vi "Main.vi"() -> ()   [LabVIEW 2013]
uses:
  source_vi/gui/type_def/device_array.ctl
  source_vi/gui/type_def/device.ctl
  source_vi/gui/type_def/general.ctl
  source_vi/gui/type_def/general_and_device.ctl
  source_vi/queues/que_enqueue_message_single.vi
  source_vi/gui/global_var.vi
panel:
  in  "config_files":string(combo) caption="Configuration file"
  out "log_bar":cluster{u8, u8}(slide) caption="Logging" scale=10.0..100.0
  out "srv_bar":cluster{u8, u8}(slide) caption="Server" scale=10.0..100.0
  in  "logging?":bool
  in  "gral_&-device":T1={"general"={"file_ext"="0.0.0.0", "TCP port"=0, "#devices"=0, "log?"=FALSE, "tcp?"=FALSE, "language"="ENG"}, "eeg_device"={"name"="", "hardware"="", "image"="", "path"=path "", "extra"="", "channels"=""}}
  out "eeg_device":T3
  in  "serving?":bool
  in  "acquiring?":bool
  in  "stopBars":bool
  out "acq_bar":cluster{u8, u8}(slide) caption="Acquistion" scale=10.0..100.0
  in  "log?":bool caption="Save Log"
  in  "tcp?":bool caption="Save Log"
  in  "refuse mrk?":bool
  out "images":picture[](array[picture])
  out "general":T2={"file_ext"="CSV", "TCP port"=0, "#devices"=0, "log?"=FALSE, "tcp?"=FALSE, "language"="ENG"}
  out "devices":T4
  in  "play?":bool
  out "log_box":string
  in  "stop?":bool
  in  "eeg_txtbox":string(combo) caption="Device"
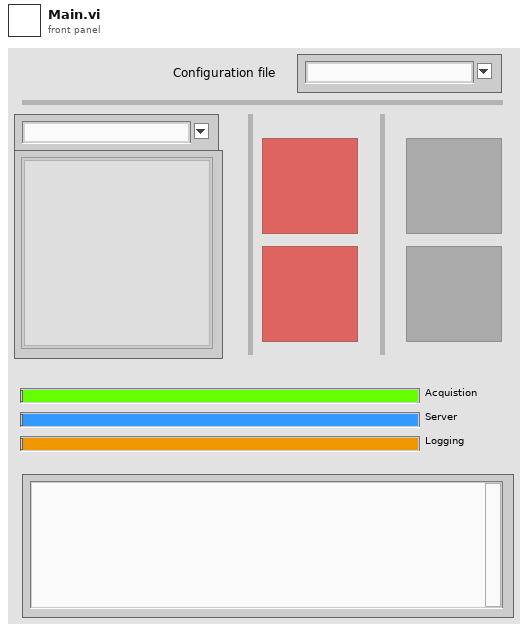
[diagram p1: front panel]
types:
  T1 = typedef "general_and_device.ctl" = cluster{"general":T2, "eeg_device":T3}
  T2 = typedef "general.ctl" = cluster{"file_ext":string, "TCP port":i32, "#devices":i32, "log?":bool, "tcp?":bool, "language":string}
  T3 = typedef "device.ctl" = cluster{"name":string, "hardware":string, "image":string, "path":path, "extra":string, "channels":string}
  T4 = typedef "device_array.ctl" = T3[]
  T5 = typedef "que_all_message_queues.ctl" = cluster{"UI":refnum<queue>, "Acquisition":refnum<queue>, "Server":refnum<queue>, "Logging":refnum<queue>}
  T6 = typedef "imagedata.ctl" = cluster{"image type":i32, "image depth":i32, "image":u8[], "mask":u8[], "colors":u32[], "Rectangle":cluster{"left":i16, "top":i16, "right":i16, "bottom":i16}}
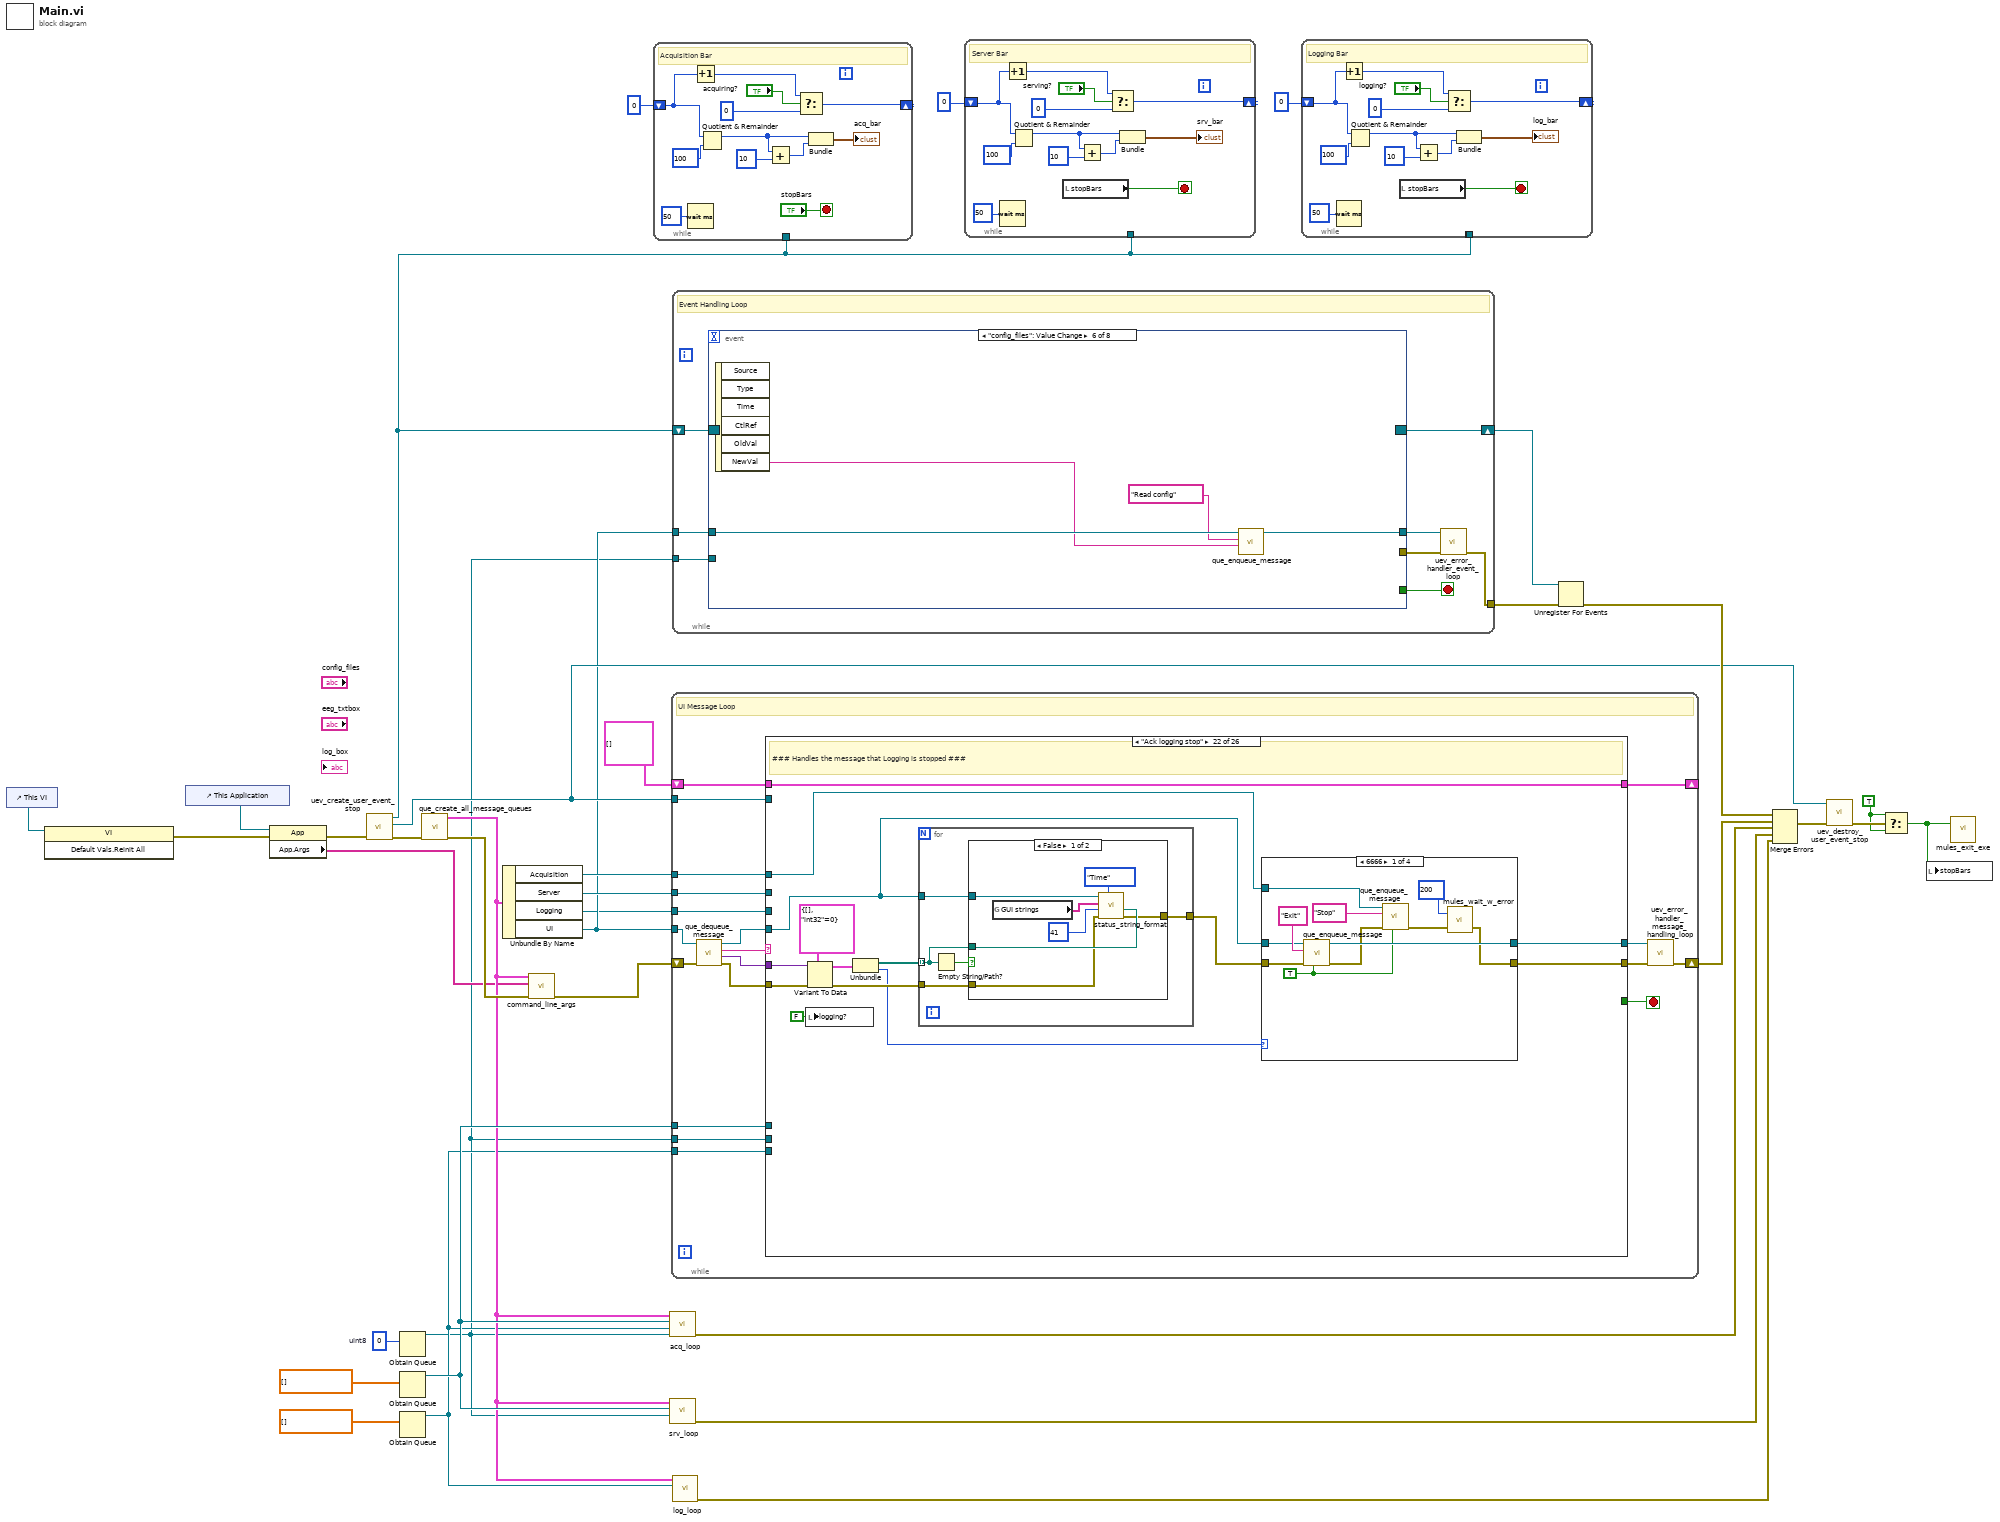
[diagram p0: block diagram]
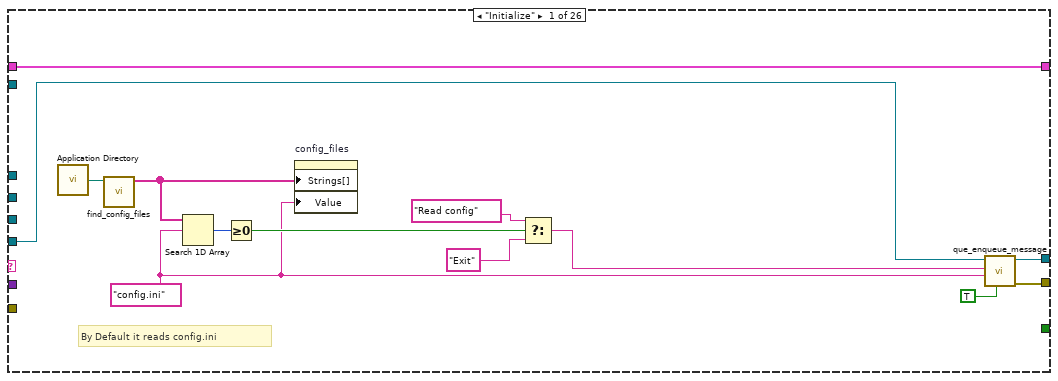
[diagram p2: hidden frame]
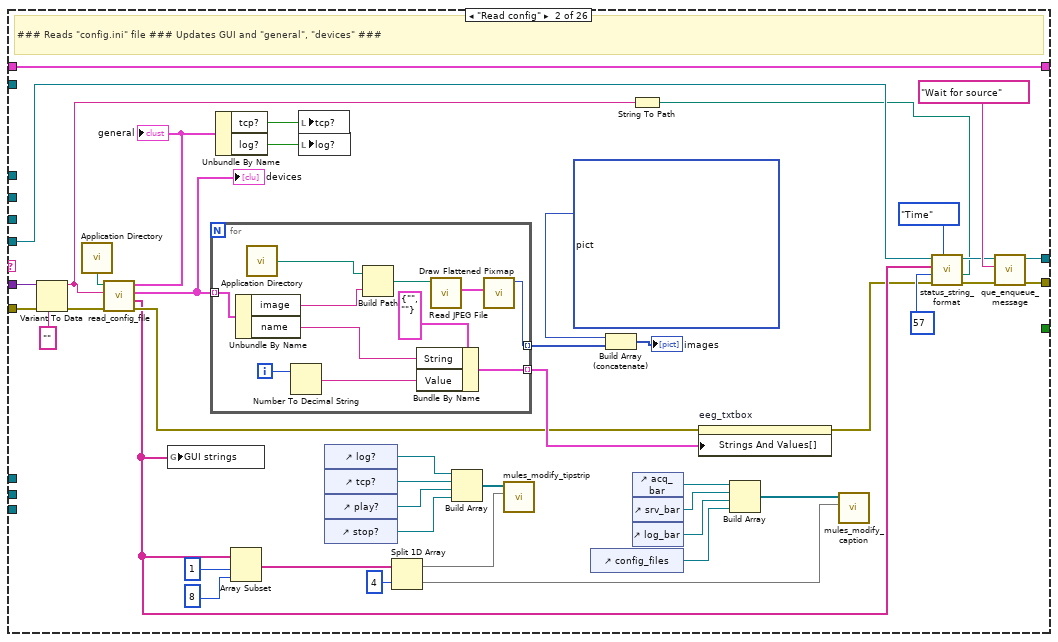
[diagram p3: hidden frame]
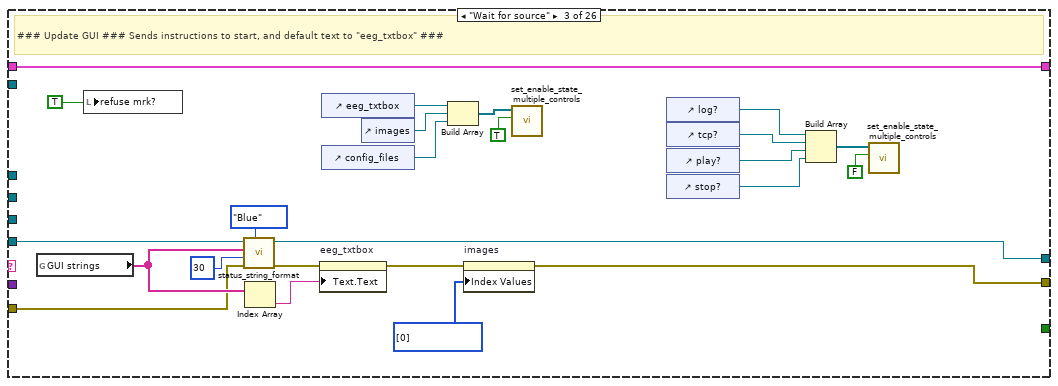
[diagram p4: hidden frame]
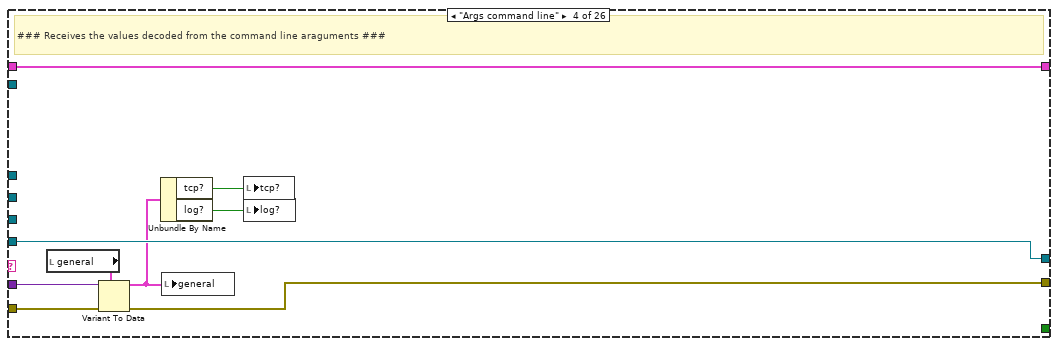
[diagram p5: hidden frame]
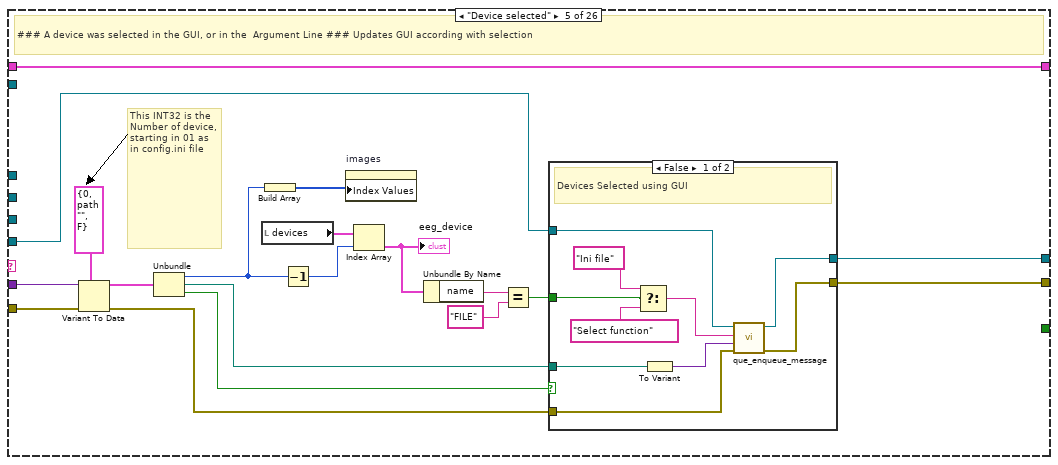
[diagram p6: hidden frame]
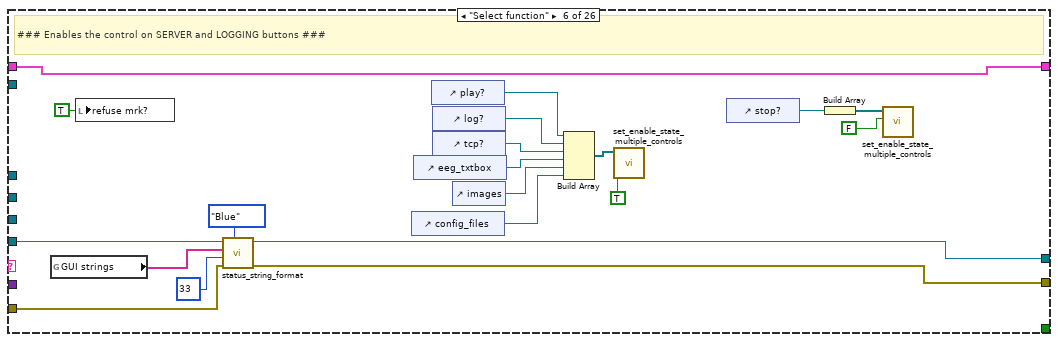
[diagram p8: hidden frame]
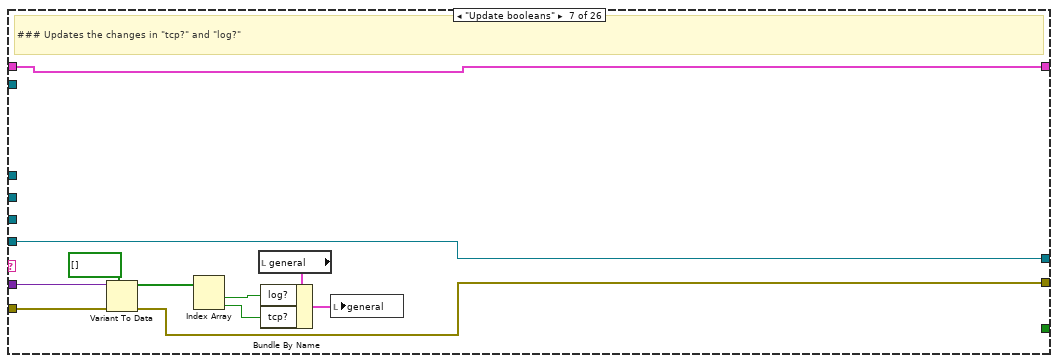
[diagram p9: hidden frame]
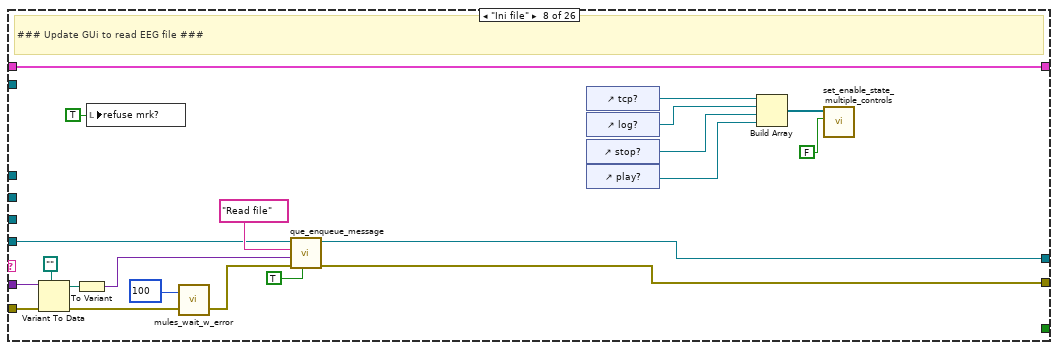
[diagram p10: hidden frame]
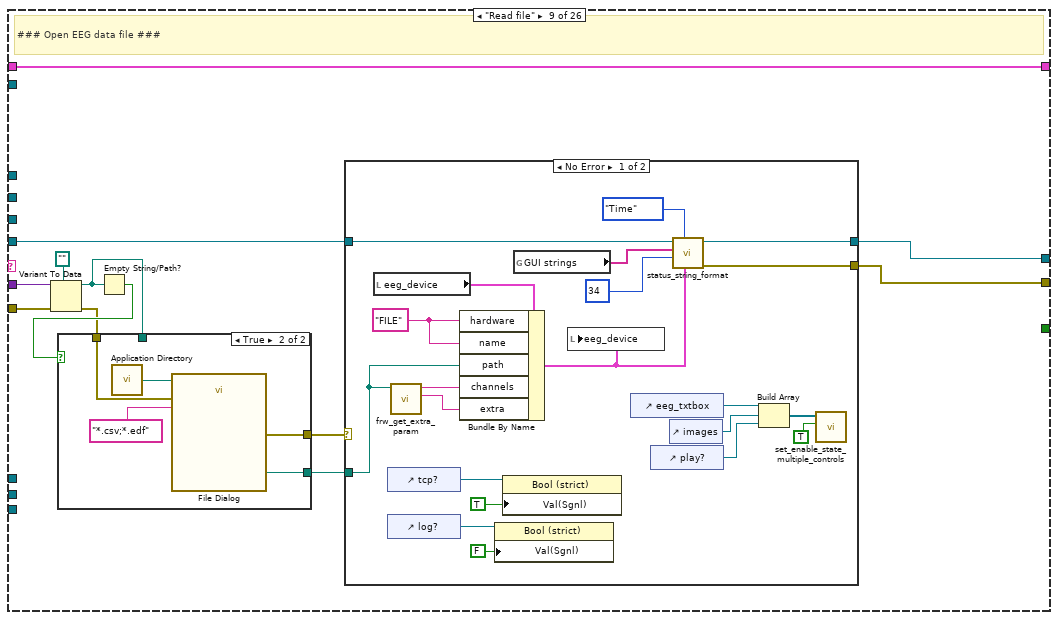
[diagram p11: hidden frame]
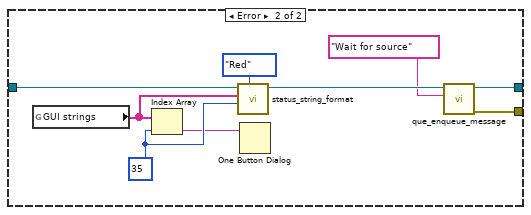
[diagram p13: hidden frame]
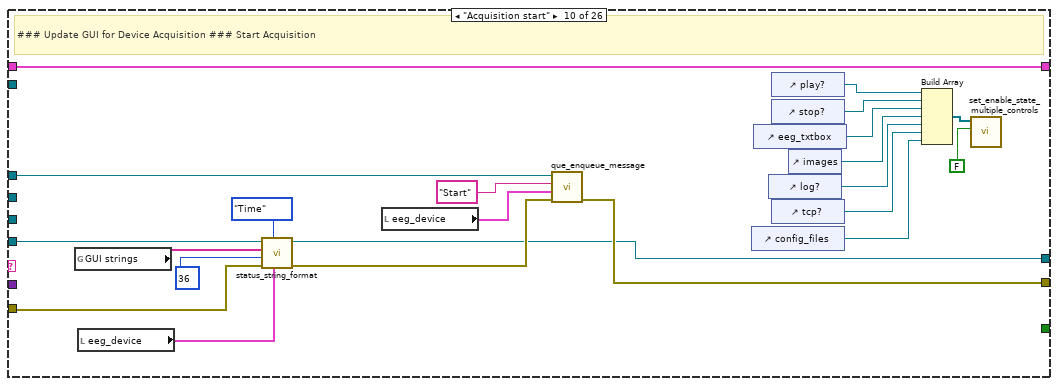
[diagram p14: hidden frame]
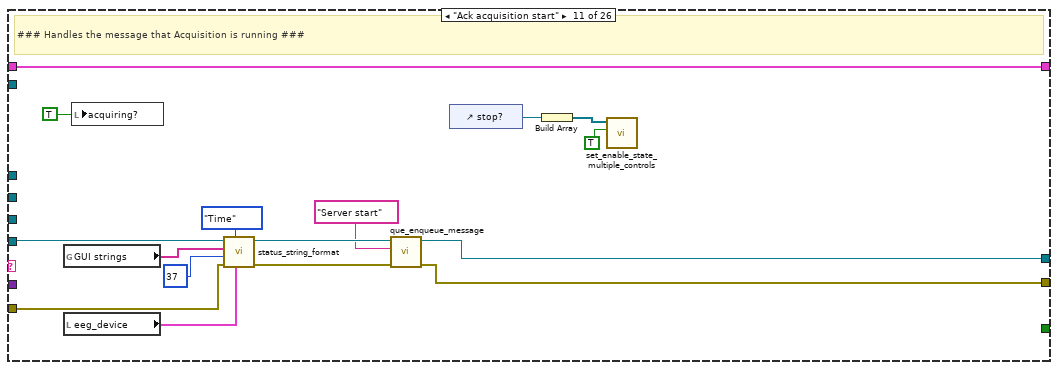
[diagram p15: hidden frame]
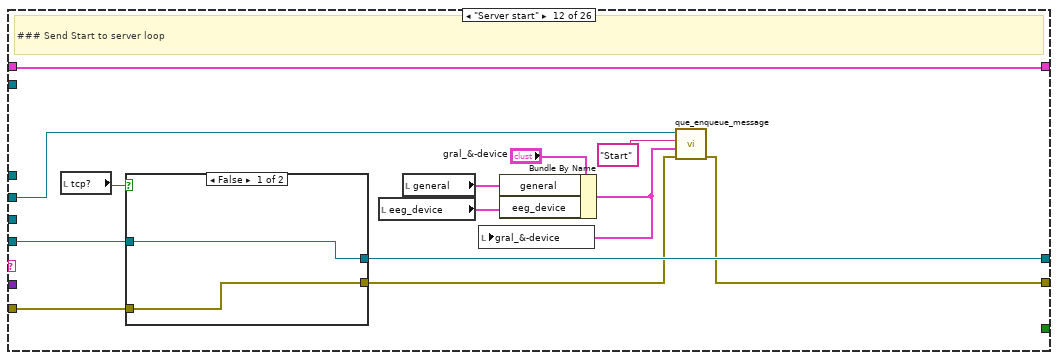
[diagram p16: hidden frame]
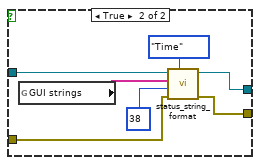
[diagram p17: hidden frame]
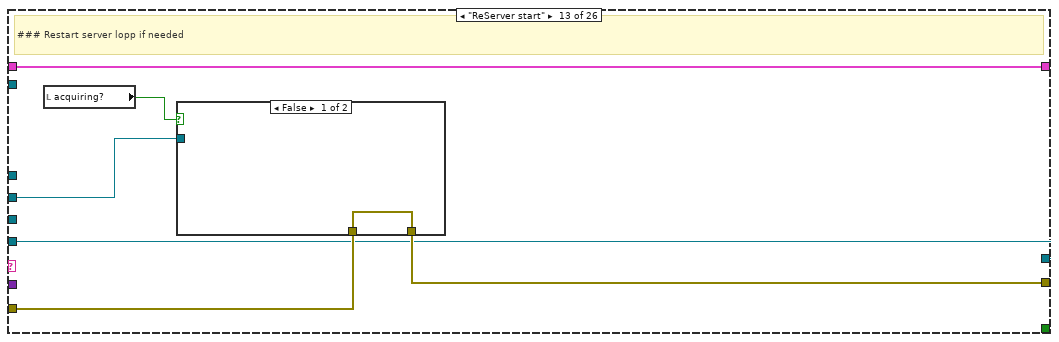
[diagram p18: hidden frame]
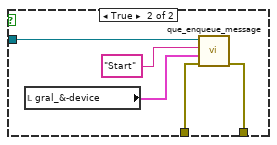
[diagram p19: hidden frame]
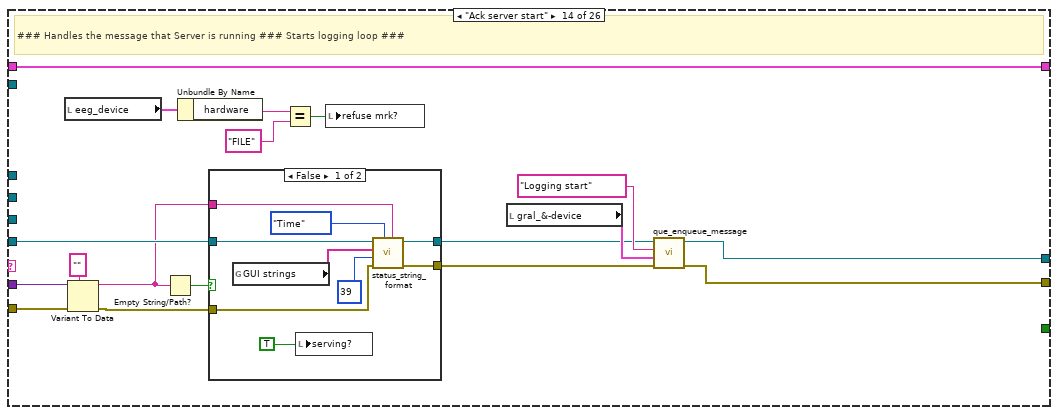
[diagram p20: hidden frame]
diagram:
  w20 = TRUE
  w27 = u8 0  # uint8
  n1 = control-ref of="This VI"() -> (w28:refnum<vi>)
  n2 = invoke class="VI" method="Default Vals.Reinit All"(reference=w28) -> (error out=w10:errorcluster)  [unwired: 2 in, 2 out]
  n3 = control-ref of="This Application"() -> (w12:refnum<vi>)
  n4 = property class="App"(reference=w12, error in=w10) -> (error out=w11:errorcluster, "App.Args"=w6:string[])  [unwired: 1 out]
  n5 = call "uev_create_user_event_stop.vi"("error in (no error)"=w11) -> ("error out"=w23:errorcluster, "User Event - Stop"=w31:refnum<user-event>, "Stop Event Registration Refnum"=w4:refnum<event-registration>)  [unwired: 8 in]
  n6 = Obtain Queue(element data type=w27) -> (queue out=w1:refnum<queue>)  [unwired: 4 in, 2 out]
  n7 = Obtain Queue(element data type=dbl[] []) -> (queue out=w16:refnum<queue>)  [unwired: 4 in, 2 out]
  n8 = Obtain Queue(element data type=dbl[] []) -> (queue out=w2:refnum<queue>)  [unwired: 4 in, 2 out]
  n9 = call "que_create_all_message_queues.vi"("error in (no error)"=w23) -> ("error out"=w8:errorcluster, "Message Queues out"=w7:T5)  [unwired: 9 in]
  n10 = Unbundle By Name(w7) -> ("Acquisition"=w30:refnum<queue>, "Server"=w29:refnum<queue>, "Logging"=w18:refnum<queue>, "UI"=w19:refnum<queue>)
  n11 = call "command_line_args.vi"("error in (no error)"=w8, "App.Args"=w6, "Message Queues"=w7) -> ("error out"=w9:errorcluster)  [unwired: 7 in, 1 out]
  n12 = while {
    shift-right: [w40] -> _
    shift-left: 0 ("y") -> [w42]
    tunnel: w4 -> [_]
    stop <- "stopBars" stop-if-true
    # "Acquisition Bar"
    n13 = Wait (ms)(milliseconds to wait=u32 50 ("millisecond multiple")) -> ()  [unwired: 1 out]
    n14 = Increment(x=w42) -> (x+1=w41:i32)
    n15 = Quotient & Remainder(x=w42, y=100) -> (x-y*floor(x/y)=w45:i32)  [unwired: 1 out]
    n16 = Add(x=w45, y=u32 10 ("millisecond multiple")) -> (x+y=w48:u32)
    n17 = Select(t=w41, s="acquiring?", f=0 ("y")) -> (s? t:f=w40:i32)
    n18 = Bundle(w45, w48) -> (→"acq_bar":cluster{i32, u32})  [unwired: 1 in]
  }
  n19 = call "acq_loop.vi"("Marker Queue"=w1, "Log queue"=w2, "Server queue"=w16, "Message Queues"=w7) -> ("error out"=w22:errorcluster)  [unwired: 7 in]
  n20 = call "srv_loop.vi"("Marker Queue"=w1, "Server queue"=w16, "Message Queues"=w7) -> ("error out"=w17:errorcluster)  [unwired: 8 in]
  n21 = while {
    tunnel: w19 -> [w66]
    shift-right: [w54] -> w32
    shift-left: w9 -> [w67]
    tunnel: w29 -> [w61]
    tunnel: w31 -> [w60]
    tunnel: w30 -> [w59]
    tunnel: w16 -> [w52]
    tunnel: w1 -> [w57]
    shift-right: [w55] -> _
    shift-left: cluster{"String":string, "Color Box":u32}[] [] -> [w56]
    tunnel: w18 -> [w53]
    tunnel: w2 -> [w50]
    stop <- w58 stop-if-true
    # "UI Message Loop"
    n22 = call "que_dequeue_message.vi"("error in (no error)"=w67, "Message Queue"=w66) -> ("error out"=w65:errorcluster, "Message Data"=w64:variant, "Message"=w49:string, "dup Message Queue"=w63:refnum<queue>)  [unwired: 6 in]
    n23 = case shown="\"Ack logging stop\"" w49 {
      selector: w49 -> [_ _ _ _ _ _ _ _ _ _ _ _ _ _ _ _ _ _ _ _ _ _ _ _ _ w701]
      tunnel: w65 -> [_ w95 w137 w164 w168 w202 w221 w235 w252 w315 w327 w342 w363 w386 w404 w415 w438 w456 w485 w508 w532 w558 w607 w666 w693 w714]
      tunnel: w64 -> [_ w96 _ w167 w181 _ w227 w236 w255 _ _ _ _ w388 _ w416 w436 w459 w484 w512 w531 w560 w622 _ w692 _]
      tunnel: w63 -> [w75 w88 w156 w162 w178 w209 w219 w238 w262 w320 w333 w345 w361 w385 w402 w412 w444 w453 w477 w509 w528 w550 _ w663 w691 w715]
      tunnel: [w80 w91 w140 w163 w177 w201 w220 w240 w257 w310 w329 w338 w362 w379 w403 w411 w440 w461 w487 w506 w530 w548 w608 w665 w690 w703] -> w62
      tunnel: w61 -> [_ _ _ _ _ _ _ _ _ _ _ w341 w364 _ _ _ _ _ w488 _ _ _ _ _ _ w712]
      tunnel: w60 -> [_ _ _ _ _ _ _ _ _ _ _ _ _ _ _ _ _ _ _ _ _ _ _ _ _ w713]
      tunnel: w59 -> [_ _ _ _ _ _ _ _ _ w312 _ _ _ _ _ _ w442 _ _ _ _ w547 _ _ _ w711]
      tunnel: [_ _ _ _ _ _ _ _ _ _ _ _ _ _ _ _ _ _ _ _ _ _ _ _ _ TRUE ("Discard?")] -> w58
      tunnel: w52 -> [_ _ _ _ _ _ _ _ _ _ _ _ _ _ _ _ _ _ _ _ _ _ _ _ _ w708]
      tunnel: w57 -> [_ _ _ _ _ _ _ _ _ _ _ _ _ _ _ _ _ _ _ _ _ _ _ _ _ w707]
      tunnel: w56 -> [w78 w116 w139 w165 w172 w214 w222 w245 w261 w321 w323 w350 w365 w389 w401 w409 w449 w475 w490 w513 w537 w559 w620 w669 w689 w699]
      tunnel: [w78 w116 w139 w165 w172 w214 w222 w245 w261 w321 w323 w350 w365 w389 w401 w409 w449 w475 w490 w513 w537 w559 w613 w669 w689 w699] -> w55
      tunnel: w53 -> [_ _ _ _ _ _ _ _ _ _ _ _ _ _ w405 _ _ _ _ _ w524 _ _ _ _ w700]
      tunnel: [w79 w90 w136 w162 w176 w200 w219 w239 w258 w309 w328 w343 w361 w372 w402 w410 w443 w457 w478 w505 w525 w549 _ w664 w686 _] -> w51
      tunnel: w50 -> [_ _ _ _ _ _ _ _ _ _ _ _ _ _ _ _ _ _ _ _ _ _ _ _ _ w704]
      frame "Initialize" {
        w70 = "config.ini" ("Message")
        # "By Default it reads config.ini"
        n24 = call <vilib>:"Application Directory.vi"() -> ("Application Directory"=w76:path)
        n25 = call "find_config_files.vi"("path"=w76) -> ("config files_names"=w73:string[])  [unwired: 10 in]
        n26 = Search 1D Array(1D array=w73, element=w70) -> (index of element=w74:i32)  [unwired: 1 in]
        n27 = Greater Or Equal To 0?(x=w74) -> (x >= 0?=w71:bool)
        n28 = property on="config_files" class="CmbBox"("Strings[]"=w73, "Value"=w70) -> ()  [unwired: 2 in, 2 out]
        n29 = Select(t="Read config" ("Message"), s=w71, f="Exit" ("Message")) -> (s? t:f=w72:string)
        n30 = call-poly "que_enqueue_message.vi"("Priority Message? (F)"=TRUE, "Message Data"=w70, "Message"=w72, "Message Queue"=w75) -> ("error out"=w80:errorcluster, "dup Message Queue"=w79:refnum<queue>)  [unwired: 6 in]
      }
      frame "Read config" {
        # "### Reads \"config.ini\" file ### Updates GUI and \"general\", \"devices\" ###"
        n31 = Variant To Data(error in=w95, type="", Variant=w96) -> (data=w85:string, error out=w94:errorcluster)
        n32 = call <vilib>:"Application Directory.vi"() -> ("Application Directory"=w98:path)
        n33 = call "read_config_file.vi"("error in (no error)"=w94, "filename"=w85, "Application Directory"=w98) -> ("error out"=w115:errorcluster, "gui_strings"=w86:string[], "devices"=w117:T4, "gral_config"=w123:T2)  [unwired: 5 in]
        "devices" <- w117
        "general" <- w123
        n34 = global write "global_var.vi" "GUI strings"(w86) -> ()
        n35 = for {
          tunnel: w117 -> [w134] mode=indexing
          tunnel: [w132] -> w121 mode=indexing
          tunnel: [w128] -> w122 mode=indexing
          i -> [w131]
          n36 = Unbundle By Name(w134) -> ("image"=w124:string, "name"=w127:string)
          n37 = call <vilib>:"Application Directory.vi"() -> ("Application Directory"=w125:path)
          n38 = Number To Decimal String(number=w131) -> (decimal integer string=w129:string)  [unwired: 1 in]
          n39 = Build Path(base path=w125, name or relative path=w124) -> (appended path=w126:path)
          n40 = Bundle By Name(cluster=cluster{"String":string, "Value":string} {"String"="", "Value"=""} ("element"), "String"=w127, "Value"=w129) -> (w128:cluster{"String":string, "Value":string})
          n41 = call <vilib>:"Read JPEG File.vi"("path to JPEG file"=w126) -> ("image data"=w133:T6)  [unwired: 8 in, 2 out]
          n42 = call <vilib>:"Draw Flattened Pixmap.vi"("image data"=w133) -> ("new picture"=w132:picture)  [unwired: 8 in]
        }
        n43 = Unbundle By Name(w123) -> ("tcp?"=w119:bool, "log?"=w118:bool)
        n44 = Array Subset(array=w86, index=1, length=8) -> (w103:string[])
        n45 = local write "tcp?"(w119) -> ()
        n46 = local write "log?"(w118) -> ()
        n47 = control-ref of="log?"() -> (w112:refnum<vi>)
        n48 = control-ref of="tcp?"() -> (w111:refnum<vi>)
        n49 = control-ref of="play?"() -> (w110:refnum<vi>)
        n50 = control-ref of="stop?"() -> (w109:refnum<vi>)
        n51 = Split 1D Array(array=w103, index=4) -> (first subarray=w101:string[], second subarray=w100:string[])
        n52 = Build Array(w112, w111, w110, w109) -> (w108:refnum<vi>[])
        n53 = call "mules_modify_tipstrip.vi"("Tip Strip Array"=w101, "Controls"=w108) -> ()  [unwired: 10 in]
        n54 = control-ref of="config_files"() -> (w93:refnum<vi>)
        n55 = Build Array (concatenate)(picture bytes[110622] ("2D Picture"), w121) -> (→"images":picture[])
        n56 = String To Path(string=w85) -> (path=w84:path)
        n57 = control-ref of="acq_bar"() -> (w107:refnum<vi>)
        n58 = control-ref of="srv_bar"() -> (w106:refnum<vi>)
        n59 = control-ref of="log_bar"() -> (w105:refnum<vi>)
        n60 = property on="eeg_txtbox" class="CmbBox"(error in=w115, "Strings And Values[]"=w122) -> (error out=w81:errorcluster)  [unwired: 1 in, 1 out]
        n61 = Build Array(w107, w106, w105, w93) -> (w104:refnum<vi>[])
        n62 = call "mules_modify_caption.vi"("Tip Strip Array"=w100, "Controls"=w104) -> ()  [unwired: 10 in]
        n63 = call "status_string_format.vi"("log_file"=w84, "color"=enum16{"Black", "Blue", "Red", "Time"}."Time", "error in (no error)"=w81, "index"=57, "gui_strings"=w86, "Message Queue"=w88) -> ("error out"=w87:errorcluster, "dup Message Queue"=w89:refnum<queue>)  [unwired: 4 in]
        n64 = call-poly "que_enqueue_message.vi"("error in (no error)"=w87, "Message"="Wait for source", "Message Queue"=w89) -> ("error out"=w91:errorcluster, "dup Message Queue"=w90:refnum<queue>)  [unwired: 7 in]
      }
      frame "Wait for source" {
        # "### Update GUI ### Sends instructions to start, and default text to \"eeg_txtbox\" ###"
        n65 = global read "global_var.vi" "GUI strings"() -> (w138:string[])
        n66 = local write "refuse mrk?"(TRUE) -> ()
        n67 = call "status_string_format.vi"("color"=enum16{"Black", "Blue", "Red", "Time"}."Blue", "error in (no error)"=w137, "index"=30, "gui_strings"=w138, "Message Queue"=w156) -> ("error out"=w152:errorcluster, "dup Message Queue"=w136:refnum<queue>)  [unwired: 5 in]
        n68 = Index Array(array=w138) -> (element=w153:string)  [unwired: 1 in]
        n69 = property on="eeg_txtbox" class="CmbBox"(error in=w152, "Text.Text"=w153) -> (error out=w155:errorcluster)  [unwired: 1 in, 1 out]
        n70 = control-ref of="eeg_txtbox"() -> (w144:refnum<vi>)
        n71 = control-ref of="config_files"() -> (w135:refnum<vi>)
        n72 = control-ref of="images"() -> (w143:refnum<vi>)
        n73 = Build Array(w144, w143, w135) -> (w141:refnum<vi>[])
        n74 = property on="images" class="Arr (strict)"(error in=w155, "Index Values"=u32[] [0]) -> (error out=w140:errorcluster)  [unwired: 1 in, 1 out]
        n75 = call "set_enable_state_multiple_controls.vi"("Enable?"=TRUE, "Controls"=w141) -> ()  [unwired: 10 in]
        n76 = control-ref of="log?"() -> (w145:refnum<vi>)
        n77 = control-ref of="tcp?"() -> (w146:refnum<vi>)
        n78 = control-ref of="play?"() -> (w147:refnum<vi>)
        n79 = control-ref of="stop?"() -> (w148:refnum<vi>)
        n80 = Build Array(w145, w146, w147, w148) -> (w151:refnum<vi>[])
        n81 = call "set_enable_state_multiple_controls.vi"("Enable?"=FALSE, "Controls"=w151) -> ()  [unwired: 10 in]
      }
      frame "Args command line" {
        # "### Receives the values decoded from the command line araguments ###"
        n82 = local read "general"() -> (w166:T2)
        n83 = Variant To Data(error in=w164, type=w166, Variant=w167) -> (data=w159:T2, error out=w163:errorcluster)
        n84 = Unbundle By Name(w159) -> ("tcp?"=w161:bool, "log?"=w160:bool)
        n85 = local write "general"(w159) -> ()
        n86 = local write "tcp?"(w161) -> ()
        n87 = local write "log?"(w160) -> ()
      }
      frame "Device selected" {
        # "This INT32 is the Number of device, starting in 01 as in config.ini file"
        # "### A device was selected in the GUI, or in the  Argument Line ### Updates GUI according with selection"
        n88 = Variant To Data(error in=w168, type=cluster{i32, path, bool} {0, path "", FALSE} ("output cluster"), Variant=w181) -> (data=w175:cluster{i32, path, bool}, error out=w169:errorcluster)
        n89 = Unbundle(w175) -> (w174:i32, w173:path, w170:bool)
        n90 = local read "devices"() -> (w182:T4)
        n91 = Build Array(w174) -> (w180:i32[])
        n92 = Decrement(x=w174) -> (x-1=w179:i32)
        n93 = property on="images" class="Arr (strict)"("Index Values"=w180) -> ()  [unwired: 2 in, 2 out]
        n94 = Index Array(array=w182, index=w179) -> (element=w183:T3)
        "eeg_device" <- w183
        n95 = Unbundle By Name(w183) -> ("name"=w184:string)
        n96 = Equal?(x=w184, y="FILE" ("Message")) -> (x = y?=w186:bool)
        n97 = case shown="False" w170 {
          tunnel: w186 -> [w193 _]
          tunnel: w178 -> [w192 w198]
          tunnel: [w191 w197] -> w177
          tunnel: [w190 w198] -> w176
          tunnel: w173 -> [w189 _]
          tunnel: w169 -> [w187 w197]
          frame False {
            # "Devices Selected using GUI"
            n98 = Select(t="Ini file" ("Message"), s=w193, f="Select function" ("Message")) -> (s? t:f=w196:string)
            n99 = To Variant(anything=w189) -> (Variant=w188:variant)
            n100 = call-poly "que_enqueue_message.vi"("error in (no error)"=w187, "Message Data"=w188, "Message"=w196, "Message Queue"=w192) -> ("error out"=w191:errorcluster, "dup Message Queue"=w190:refnum<queue>)  [unwired: 6 in]
          }
          frame True {
            # "Device Selected in Argument Line"
          }
        }
      }
      frame "Select function" {
        # "### Enables the control on SERVER and LOGGING buttons ###"
        n101 = global read "global_var.vi" "GUI strings"() -> (w208:string[])
        n102 = local write "refuse mrk?"(TRUE) -> ()
        n103 = call "status_string_format.vi"("color"=enum16{"Black", "Blue", "Red", "Time"}."Blue", "error in (no error)"=w202, "index"=33, "gui_strings"=w208, "Message Queue"=w209) -> ("error out"=w201:errorcluster, "dup Message Queue"=w200:refnum<queue>)  [unwired: 5 in]
        n104 = control-ref of="config_files"() -> (w199:refnum<vi>)
        n105 = control-ref of="eeg_txtbox"() -> (w211:refnum<vi>)
        n106 = control-ref of="play?"() -> (w203:refnum<vi>)
        n107 = control-ref of="log?"() -> (w204:refnum<vi>)
        n108 = control-ref of="tcp?"() -> (w205:refnum<vi>)
        n109 = control-ref of="images"() -> (w210:refnum<vi>)
        n110 = Build Array(w203, w204, w205, w211, w210, w199) -> (w213:refnum<vi>[])
        n111 = call "set_enable_state_multiple_controls.vi"("Enable?"=TRUE, "Controls"=w213) -> ()  [unwired: 10 in]
        n112 = control-ref of="stop?"() -> (w218:refnum<vi>)
        n113 = Build Array(w218) -> (w217:refnum<vi>[])
        n114 = call "set_enable_state_multiple_controls.vi"("Enable?"=FALSE, "Controls"=w217) -> ()  [unwired: 10 in]
      }
      frame "Update booleans" {
        # "### Updates the changes in \"tcp?\" and \"log?\""
        n115 = Variant To Data(error in=w221, type=bool[] [], Variant=w227) -> (data=w225:bool[], error out=w220:errorcluster)
        n116 = Index Array(array=w225) -> (element #1=w224:bool, element #2=w223:bool)  [unwired: 2 in]
        n117 = local read "general"() -> (w228:T2)
        n118 = Bundle By Name(cluster=w228, "log?"=w224, "tcp?"=w223) -> (w229:T2)
        n119 = local write "general"(w229) -> ()
      }
      frame "Ini file" {
        # "### Update GUi to read EEG file ###"
        n120 = Variant To Data(error in=w235, type=path "", Variant=w236) -> (data=w232:path, error out=w234:errorcluster)
        n121 = To Variant(anything=w232) -> (Variant=w231:variant)
        n122 = local write "refuse mrk?"(TRUE) -> ()
        n123 = call "mules_wait_w_error.vi"("error in (no error)"=w234, "milliseconds to wait"=u32 100) -> ("error out"=w242:errorcluster)  [unwired: 1 in]
        n124 = call-poly "que_enqueue_message.vi"("Priority Message? (F)"=TRUE, "error in (no error)"=w242, "Message Data"=w231, "Message"="Read file", "Message Queue"=w238) -> ("error out"=w240:errorcluster, "dup Message Queue"=w239:refnum<queue>)  [unwired: 5 in]
        n125 = control-ref of="tcp?"() -> (w237:refnum<vi>)
        n126 = control-ref of="log?"() -> (w244:refnum<vi>)
        n127 = control-ref of="stop?"() -> (w250:refnum<vi>)
        n128 = control-ref of="play?"() -> (w249:refnum<vi>)
        n129 = Build Array(w237, w244, w250, w249) -> (w248:refnum<vi>[])
        n130 = call "set_enable_state_multiple_controls.vi"("Enable?"=FALSE, "Controls"=w248) -> ()  [unwired: 10 in]
      }
      frame "Read file" {
        # "### Open EEG data file ###"
        n131 = Variant To Data(error in=w252, type=path "", Variant=w255) -> (data=w253:path, error out=w251:errorcluster)
        n132 = Empty String/Path?(string/path=w253) -> (empty?=w254:bool)
        n133 = case shown="True" w254 {
          tunnel: [w263 w269] -> w260
          tunnel: [w264 w268] -> w259
          tunnel: w253 -> [w264 _]
          tunnel: w251 -> [w263 w267]
          frame False {
          }
          frame True {
            n134 = call <vilib>:"Application Directory.vi"() -> ("Application Directory"=w265:path)
            n135 = call "File Dialog"("start path"=w265, "error in"=w267, "pattern (all files)"="*.csv;*.edf") -> ("selected path"=w268:path, "error out"=w269:errorcluster)  [unwired: 9 in, 2 out]
          }
        }
        n136 = case shown="No Error" w260 {
          tunnel: w262 -> [w286 w299]
          tunnel: w259 -> [w283 _]
          tunnel: [w287 w294] -> w258
          tunnel: [w279 w292] -> w257
          frame No Error {
            w280 = "FILE" ("Message")
            n137 = local read "eeg_device"() -> (w290:T3)
            n138 = control-ref of="tcp?"() -> (w270:refnum<vi>)
            n139 = control-ref of="log?"() -> (w273:refnum<vi>)
            n140 = call "frw_get_extra_param.vi"("Path"=w283) -> ("extra_string"=w281:string, "channels_str"=w282:string)  [unwired: 9 in]
            n141 = Bundle By Name(cluster=w290, "hardware"=w280, "name"=w280, "path"=w283, "channels"=w282, "extra"=w281) -> (w285:T3)
            n142 = property class="Bool (strict)"(reference=w273, "Val(Sgnl)"=FALSE ("Value (Signaling)")) -> ()  [unwired: 1 in, 2 out]
            n143 = property class="Bool (strict)"(reference=w270, "Val(Sgnl)"=TRUE ("Value (Signaling)")) -> ()  [unwired: 1 in, 2 out]
            n144 = global read "global_var.vi" "GUI strings"() -> (w289:string[])
            n145 = local write "eeg_device"(w285) -> ()
            n146 = control-ref of="eeg_txtbox"() -> (w275:refnum<vi>)
            n147 = control-ref of="play?"() -> (w277:refnum<vi>)
            n148 = control-ref of="images"() -> (w274:refnum<vi>)
            n149 = call "status_string_format.vi"("eeg_device"=w285, "color"=enum16{"Black", "Blue", "Red", "Time"}."Time", "index"=34, "gui_strings"=w289, "Message Queue"=w286) -> ("error out"=w279:errorcluster, "dup Message Queue"=w287:refnum<queue>)  [unwired: 5 in]
            n150 = Build Array(w275, w274, w277) -> (w276:refnum<vi>[])
            n151 = call "set_enable_state_multiple_controls.vi"("Enable?"=TRUE, "Controls"=w276) -> ()  [unwired: 10 in]
          }
          frame Error {
            w297 = 35 ("index")
            n152 = global read "global_var.vi" "GUI strings"() -> (w298:string[])
            n153 = Index Array(array=w298, index=w297) -> (element=w291:string)
            n154 = call "status_string_format.vi"("color"=enum16{"Black", "Blue", "Red", "Time"}."Red", "index"=w297, "gui_strings"=w298, "Message Queue"=w299) -> ("dup Message Queue"=w295:refnum<queue>)  [unwired: 6 in, 1 out]
            n155 = One Button Dialog(message=w291) -> ()  [unwired: 1 in, 1 out]
            n156 = call-poly "que_enqueue_message.vi"("Message"="Wait for source", "Message Queue"=w295) -> ("error out"=w292:errorcluster, "dup Message Queue"=w294:refnum<queue>)  [unwired: 8 in]
          }
        }
      }
      frame "Acquisition start" {
        # "### Update GUI for Device Acquisition ### Start Acquisition"
        n157 = global read "global_var.vi" "GUI strings"() -> (w319:string[])
        n158 = local read "eeg_device"() -> (w316:T3)
        n159 = call "status_string_format.vi"("eeg_device"=w316, "color"=enum16{"Black", "Blue", "Red", "Time"}."Time", "error in (no error)"=w315, "index"=36, "gui_strings"=w319, "Message Queue"=w320) -> ("error out"=w311:errorcluster, "dup Message Queue"=w309:refnum<queue>)  [unwired: 4 in]
        n160 = local read "eeg_device"() -> (w313:T3)
        n161 = call-poly "que_enqueue_message.vi"("error in (no error)"=w311, "Message Data"=w313, "Message"="Start", "Message Queue"=w312) -> ("error out"=w310:errorcluster)  [unwired: 6 in, 1 out]
        n162 = control-ref of="config_files"() -> (w300:refnum<vi>)
        n163 = control-ref of="eeg_txtbox"() -> (w304:refnum<vi>)
        n164 = control-ref of="log?"() -> (w302:refnum<vi>)
        n165 = control-ref of="play?"() -> (w308:refnum<vi>)
        n166 = control-ref of="stop?"() -> (w307:refnum<vi>)
        n167 = control-ref of="tcp?"() -> (w301:refnum<vi>)
        n168 = control-ref of="images"() -> (w303:refnum<vi>)
        n169 = Build Array(w308, w307, w304, w303, w302, w301, w300) -> (w306:refnum<vi>[])
        n170 = call "set_enable_state_multiple_controls.vi"("Enable?"=FALSE, "Controls"=w306) -> ()  [unwired: 10 in]
      }
      frame "Ack acquisition start" {
        # "### Handles the message that Acquisition is running ###"
        n171 = global read "global_var.vi" "GUI strings"() -> (w337:string[])
        n172 = local read "eeg_device"() -> (w334:T3)
        n173 = local write "acquiring?"(TRUE ("runBar1?")) -> ()
        n174 = call "status_string_format.vi"("eeg_device"=w334, "color"=enum16{"Black", "Blue", "Red", "Time"}."Time", "error in (no error)"=w327, "index"=37, "gui_strings"=w337, "Message Queue"=w333) -> ("error out"=w330:errorcluster, "dup Message Queue"=w332:refnum<queue>)  [unwired: 4 in]
        n175 = call-poly "que_enqueue_message.vi"("error in (no error)"=w330, "Message"="Server start", "Message Queue"=w332) -> ("error out"=w329:errorcluster, "dup Message Queue"=w328:refnum<queue>)  [unwired: 7 in]
        n176 = control-ref of="stop?"() -> (w326:refnum<vi>)
        n177 = Build Array(w326) -> (w325:refnum<vi>[])
        n178 = call "set_enable_state_multiple_controls.vi"("Enable?"=TRUE, "Controls"=w325) -> ()  [unwired: 10 in]
      }
      frame "Server start" {
        # "### Send Start to server loop"
        n179 = local read "tcp?"() -> (w344:bool)
        n180 = case shown="False" w344 {
          tunnel: w345 -> [w351 w356]
          tunnel: w342 -> [w352 w355]
          tunnel: [w351 w354] -> w343
          tunnel: [w352 w353] -> w339
          frame False {
          }
          frame True {
            n181 = global read "global_var.vi" "GUI strings"() -> (w358:string[])
            n182 = call "status_string_format.vi"("color"=enum16{"Black", "Blue", "Red", "Time"}."Time", "error in (no error)"=w355, "index"=38, "gui_strings"=w358, "Message Queue"=w356) -> ("error out"=w353:errorcluster, "dup Message Queue"=w354:refnum<queue>)  [unwired: 5 in]
          }
        }
        n183 = local read "eeg_device"() -> (w346:T3)
        n184 = local read "general"() -> (w347:T2)
        n185 = Bundle By Name(cluster="gral_&-device", "general"=w347, "eeg_device"=w346) -> (w340:T1)
        n186 = local write "gral_&-device"(w340) -> ()
        n187 = call-poly "que_enqueue_message.vi"("error in (no error)"=w339, "Message Data"=w340, "Message"="Start", "Message Queue"=w341) -> ("error out"=w338:errorcluster)  [unwired: 6 in, 1 out]
      }
      frame "ReServer start" {
        # "### Restart server lopp if needed"
        n188 = local read "acquiring?"() -> (w360:bool)
        n189 = case shown="False" w360 {
          tunnel: w364 -> [_ w370]
          tunnel: w363 -> [w366 w368]
          tunnel: [w366 w367] -> w362
          frame False {
          }
          frame True {
            n190 = local read "gral_&-device"() -> (w369:T1)
            n191 = call-poly "que_enqueue_message.vi"("error in (no error)"=w368, "Message Data"=w369, "Message"="Start", "Message Queue"=w370) -> ("error out"=w367:errorcluster)  [unwired: 6 in, 1 out]
          }
        }
      }
      frame "Ack server start" {
        # "### Handles the message that Server is running ### Starts logging loop ###"
        n192 = local read "eeg_device"() -> (w377:T3)
        n193 = Variant To Data(error in=w386, type="" ("String"), Variant=w388) -> (data=w381:string, error out=w378:errorcluster)
        n194 = Empty String/Path?(string/path=w381) -> (empty?=w382:bool)
        n195 = Unbundle By Name(w377) -> ("hardware"=w376:string)
        n196 = case shown="False" w382 {
          tunnel: w385 -> [w398 w399]
          tunnel: w381 -> [w394 _]
          tunnel: [w393 w400] -> w380
          tunnel: w378 -> [w392 w400]
          tunnel: [w391 w399] -> w373
          frame False {
            n197 = global read "global_var.vi" "GUI strings"() -> (w397:string[])
            n198 = local write "serving?"(TRUE ("runBar1?")) -> ()
            n199 = call "status_string_format.vi"("ip"=w394, "color"=enum16{"Black", "Blue", "Red", "Time"}."Time", "error in (no error)"=w392, "index"=39, "gui_strings"=w397, "Message Queue"=w398) -> ("error out"=w393:errorcluster, "dup Message Queue"=w391:refnum<queue>)  [unwired: 4 in]
          }
          frame True {
          }
        }
        n200 = Equal?(x=w376, y="FILE") -> (x = y?=w374:bool)
        n201 = local write "refuse mrk?"(w374) -> ()
        n202 = local read "gral_&-device"() -> (w383:T1)
        n203 = call-poly "que_enqueue_message.vi"("error in (no error)"=w380, "Message Data"=w383, "Message"="Logging start", "Message Queue"=w373) -> ("error out"=w379:errorcluster, "dup Message Queue"=w372:refnum<queue>)  [unwired: 6 in]
      }
      frame "Logging start" {
        n204 = local read "gral_&-device"() -> (w406:T1)
        n205 = call-poly "que_enqueue_message.vi"("error in (no error)"=w404, "Message Data"=w406, "Message"="Start", "Message Queue"=w405) -> ("error out"=w403:errorcluster)  [unwired: 6 in, 1 out]
      }
      frame "Ack logging start" {
        n206 = Variant To Data(error in=w415, type=path[] [], Variant=w416) -> (data=w414:path[], error out=w413:errorcluster)
        n207 = for {
          tunnel: w414 -> [w421] mode=indexing
          tunnel: w412 -> [w422]
          tunnel: [w420] -> w411
          tunnel: w413 -> [w419]
          tunnel: [w418] -> w410
          n208 = Empty String/Path?(string/path=w421) -> (empty?=w423:bool)
          n209 = case shown="False" w423 {
            tunnel: w422 -> [w430 w432]
            tunnel: w421 -> [w429 _]
            tunnel: [w426 w433] -> w420
            tunnel: w419 -> [w425 w433]
            tunnel: [w424 w432] -> w418
            frame False {
              n210 = global read "global_var.vi" "GUI strings"() -> (w431:string[])
              n211 = call "status_string_format.vi"("log_file"=w429, "color"=enum16{"Black", "Blue", "Red", "Time"}."Time", "error in (no error)"=w425, "index"=53, "gui_strings"=w431, "Message Queue"=w430) -> ("error out"=w426:errorcluster, "dup Message Queue"=w424:refnum<queue>)  [unwired: 4 in]
            }
            frame True {
            }
          }
        }
        n212 = local read "log?"() -> (w408:bool)
        n213 = local write "logging?"(w408) -> ()
      }
      frame "Acquisition stop" {
        w439 = 0  # int32
        # "### Stops Acquisition ###"
        n214 = Variant To Data(error in=w438, type=w439, Variant=w436) -> (data=w434:i32, error out=w437:errorcluster)
        n215 = To Variant(anything=w434) -> (Variant=w435:variant)
        n216 = global read "global_var.vi" "GUI strings"() -> (w448:string[])
        n217 = local read "eeg_device"() -> (w445:T3)
        n218 = call "status_string_format.vi"("eeg_device"=w445, "color"=enum16{"Black", "Blue", "Red", "Time"}."Time", "error in (no error)"=w437, "index"=45, "gui_strings"=w448, "Message Queue"=w444) -> ("error out"=w441:errorcluster, "dup Message Queue"=w443:refnum<queue>)  [unwired: 4 in]
        n219 = call-poly "que_enqueue_message.vi"("error in (no error)"=w441, "Message Data"=w435, "Message"="Stop", "Message Queue"=w442) -> ("error out"=w440:errorcluster)  [unwired: 6 in, 1 out]
      }
      frame "Ack acquisition stop" {
        w458 = 0  # int32
        # "### Handles the message that Acquisition is stopped ###"
        n220 = Variant To Data(error in=w456, type=w458, Variant=w459) -> (data=w455:i32, error out=w452:errorcluster)
        n221 = local write "acquiring?"(FALSE ("runBar1?")) -> ()
        n222 = global read "global_var.vi" "GUI strings"() -> (w464:string[])
        n223 = local read "eeg_device"() -> (w466:T3)
        n224 = call "status_string_format.vi"("eeg_device"=w466, "color"=enum16{"Black", "Blue", "Red", "Time"}."Time", "error in (no error)"=w452, "index"=46, "gui_strings"=w464, "Message Queue"=w453) -> ("dup Message Queue"=w454:refnum<queue>)  [unwired: 4 in, 1 out]
        n225 = To Variant(anything=w455) -> (Variant=w460:variant)
        n226 = call-poly "que_enqueue_message.vi"("Message Data"=w460, "Message"="Server stop", "Message Queue"=w454) -> ("error out"=w461:errorcluster, "dup Message Queue"=w457:refnum<queue>)  [unwired: 7 in]
        n227 = control-ref of="config_files"() -> (w451:refnum<vi>)
        n228 = control-ref of="eeg_txtbox"() -> (w470:refnum<vi>)
        n229 = control-ref of="log?"() -> (w468:refnum<vi>)
        n230 = control-ref of="play?"() -> (w474:refnum<vi>)
        n231 = control-ref of="stop?"() -> (w473:refnum<vi>)
        n232 = control-ref of="tcp?"() -> (w467:refnum<vi>)
        n233 = control-ref of="images"() -> (w469:refnum<vi>)
        n234 = Build Array(w451, w474, w473, w470, w469, w468, w467) -> (w472:refnum<vi>[])
        n235 = call "set_enable_state_multiple_controls.vi"("Enable?"=FALSE, "Controls"=w472) -> ()  [unwired: 10 in]
      }
      frame "Server stop" {
        w486 = 0  # int32
        n236 = Variant To Data(error in=w485, type=w486, Variant=w484) -> (data=w482:i32, error out=w480:errorcluster)
        n237 = local read "tcp?"() -> (w481:bool)
        n238 = case shown="True" w481 {
          tunnel: w477 -> [w492 w496]
          tunnel: [w491 w495] -> w479
          tunnel: [w492 w494] -> w478
          tunnel: w480 -> [w491 w493]
          frame False {
          }
          frame True {
            n239 = global read "global_var.vi" "GUI strings"() -> (w497:string[])
            n240 = call "status_string_format.vi"("color"=enum16{"Black", "Blue", "Red", "Time"}."Time", "error in (no error)"=w493, "index"=54, "gui_strings"=w497, "Message Queue"=w496) -> ("error out"=w495:errorcluster, "dup Message Queue"=w494:refnum<queue>)  [unwired: 5 in]
          }
        }
        n241 = To Variant(anything=w482) -> (Variant=w483:variant)
        n242 = call-poly "que_enqueue_message.vi"("error in (no error)"=w479, "Message Data"=w483, "Message"="Stop", "Message Queue"=w488) -> ("error out"=w487:errorcluster)  [unwired: 6 in, 1 out]
      }
      frame "Ack server stop" {
        w511 = 0  # Int32
        # "### Handles the message that Server is stopped ###"
        n243 = Variant To Data(error in=w508, type=w511, Variant=w512) -> (data=w510:i32, error out=w507:errorcluster)
        n244 = local write "serving?"(FALSE ("runBar1?")) -> ()
        n245 = local read "tcp?"() -> (w503:bool)
        n246 = case shown="True" w503 {
          tunnel: w509 -> [w516 w520]
          tunnel: [w515 w519] -> w501
          tunnel: [w516 w518] -> w502
          tunnel: w507 -> [w515 w517]
          frame False {
          }
          frame True {
            n247 = global read "global_var.vi" "GUI strings"() -> (w521:string[])
            n248 = call "status_string_format.vi"("color"=enum16{"Black", "Blue", "Red", "Time"}."Time", "error in (no error)"=w517, "index"=40, "gui_strings"=w521, "Message Queue"=w520) -> ("error out"=w519:errorcluster, "dup Message Queue"=w518:refnum<queue>)  [unwired: 5 in]
          }
        }
        n249 = To Variant(anything=w510) -> (Variant=w500:variant)
        n250 = call-poly "que_enqueue_message.vi"("error in (no error)"=w501, "Message Data"=w500, "Message"="Logging stop", "Message Queue"=w502) -> ("error out"=w506:errorcluster, "dup Message Queue"=w505:refnum<queue>)  [unwired: 6 in]
      }
      frame "Logging stop" {
        w535 = 0  # int32
        n251 = Variant To Data(error in=w532, type=w535, Variant=w531) -> (data=w533:i32, error out=w529:errorcluster)
        n252 = local read "log?"() -> (w527:bool)
        n253 = case shown="True" w527 {
          tunnel: w528 -> [w539 w543]
          tunnel: [w538 w542] -> w526
          tunnel: [w539 w541] -> w525
          tunnel: w529 -> [w538 w540]
          frame False {
          }
          frame True {
            n254 = global read "global_var.vi" "GUI strings"() -> (w544:string[])
            n255 = call "status_string_format.vi"("color"=enum16{"Black", "Blue", "Red", "Time"}."Time", "error in (no error)"=w540, "index"=55, "gui_strings"=w544, "Message Queue"=w543) -> ("error out"=w542:errorcluster, "dup Message Queue"=w541:refnum<queue>)  [unwired: 5 in]
          }
        }
        n256 = To Variant(anything=w533) -> (Variant=w534:variant)
        n257 = call-poly "que_enqueue_message.vi"("error in (no error)"=w526, "Message Data"=w534, "Message"="Stop", "Message Queue"=w524) -> ("error out"=w530:errorcluster)  [unwired: 6 in, 1 out]
      }
      frame "Ack logging stop" {
        # "### Handles the message that Logging is stopped ###"
        n258 = local write "logging?"(FALSE ("runBar1?")) -> ()
        n259 = Variant To Data(error in=w558, type=cluster{path[], "int32":i32} {[], "int32"=0} ("output cluster"), Variant=w560) -> (data=w554:cluster{path[], "int32":i32}, error out=w557:errorcluster)
        n260 = Unbundle(w554) -> (w553:path[], "int32"=w552:i32)
        n261 = for {
          tunnel: w553 -> [w595] mode=indexing
          tunnel: w550 -> [w596]
          tunnel: [w594] -> w551
          tunnel: w557 -> [w593]
          n262 = Empty String/Path?(string/path=w595) -> (empty?=w597:bool)
          n263 = case shown="False" w597 {
            tunnel: w596 -> [w603 _]
            tunnel: w595 -> [w602 _]
            tunnel: [w599 w605] -> w594
            tunnel: w593 -> [w598 w605]
            frame False {
              n264 = global read "global_var.vi" "GUI strings"() -> (w604:string[])
              n265 = call "status_string_format.vi"("log_file"=w602, "color"=enum16{"Black", "Blue", "Red", "Time"}."Time", "error in (no error)"=w598, "index"=41, "gui_strings"=w604, "Message Queue"=w603) -> ("error out"=w599:errorcluster)  [unwired: 4 in, 1 out]
            }
            frame True {
            }
          }
        }
        n266 = case shown="6666" w552 {
          tunnel: w551 -> [w570 w575 w583 w589]
          tunnel: w550 -> [w569 w578 w586 w592]
          tunnel: [w568 w582 w585 w591] -> w549
          tunnel: [w562 w581 w584 w590] -> w548
          tunnel: w547 -> [w564 _ _ _]
          frame 6666 {
            w566 = TRUE ("Priority Message? (F)")
            n267 = call-poly "que_enqueue_message.vi"("Priority Message? (F)"=w566, "error in (no error)"=w570, "Message"="Exit", "Message Queue"=w569) -> ("error out"=w567:errorcluster, "dup Message Queue"=w568:refnum<queue>)  [unwired: 6 in]
            n268 = call-poly "que_enqueue_message.vi"("Priority Message? (F)"=w566, "error in (no error)"=w567, "Message"="Stop", "Message Queue"=w564) -> ("error out"=w563:errorcluster)  [unwired: 6 in, 1 out]
            n269 = call "mules_wait_w_error.vi"("error in (no error)"=w563, "milliseconds to wait"=u32 200) -> ("error out"=w562:errorcluster)  [unwired: 1 in]
          }
          frame 3 {
            n270 = local read "eeg_device"() -> (w573:T3)
            n271 = global read "global_var.vi" "GUI strings"() -> (w577:string[])
            n272 = call "status_string_format.vi"("eeg_device"=w573, "color"=enum16{"Black", "Blue", "Red", "Time"}."Time", "error in (no error)"=w575, "index"=56, "gui_strings"=w577, "Message Queue"=w578) -> ("error out"=w574:errorcluster, "dup Message Queue"=w580:refnum<queue>)  [unwired: 4 in]
            n273 = call-poly "que_enqueue_message.vi"("error in (no error)"=w574, "Message"="Wait for source", "Message Queue"=w580) -> ("error out"=w581:errorcluster, "dup Message Queue"=w582:refnum<queue>)  [unwired: 7 in]
          }
          frame 1, Default {
            n274 = call-poly "que_enqueue_message.vi"("error in (no error)"=w583, "Message"="Wait for source", "Message Queue"=w586) -> ("error out"=w584:errorcluster, "dup Message Queue"=w585:refnum<queue>)  [unwired: 7 in]
          }
          frame 66 {
            n275 = call-poly "que_enqueue_message.vi"("error in (no error)"=w589, "Message"="Server start", "Message Queue"=w592) -> ("error out"=w590:errorcluster, "dup Message Queue"=w591:refnum<queue>)  [unwired: 7 in]
          }
        }
      }
      frame "WriteConsole" {
        # "### Writes a text in the Console-like text box, each line have its own color  ###"
        n276 = Variant To Data(error in=w607, type="", Variant=w622) -> (data=w619:string)  [unwired: 1 out]
        n277 = Search/Split String(string=w619, offset (0)=1 ("length (rest)")) -> (substring before match=w617:string, match + rest of string=w616:string)  [unwired: 1 in, 1 out]
        n278 = case shown="\"T\"" w617 {
          tunnel: w616 -> [w639 w648 w654 w660]
          tunnel: cluster{"String":string, "Color Box":u32} {"String"="", "Color Box"=16860} ("Cluster") -> [w637 w646 w652 w658]
          tunnel: [w636 w645 w651 w657] -> w606
          frame "T" {
            w642 = TRUE ("time colon?")
            n279 = call "mules_date2string.vi"("time colon?"=w642, "seconds?"=w642) -> ("time_string"=w641:string)  [unwired: 7 in, 2 out]
            n280 = call <vilib>:"Space Constant.vi"() -> ("String"=w640:string)
            n281 = Concatenate Strings(w641, w640, w639, "\r\n") -> (w638:string)
            n282 = Bundle(cluster=w637, "String"=w638, "Color Box"=u32 16777222) -> (w636:cluster{"String":string, "Color Box":u32})
          }
          frame "B" {
            n283 = Concatenate Strings(w648, "\r\n") -> (w644:string)
            n284 = Bundle(cluster=w646, "String"=w644, "Color Box"=u32 16860) -> (w645:cluster{"String":string, "Color Box":u32})
          }
          frame "K", Default {
            n285 = Concatenate Strings(w654, "\r\n") -> (w650:string)
            n286 = Bundle(cluster=w652, "String"=w650, "Color Box"=u32 16777222) -> (w651:cluster{"String":string, "Color Box":u32})
          }
          frame "R" {
            n287 = Concatenate Strings(w660, "\r\n") -> (w656:string)
            n288 = Bundle(cluster=w658, "String"=w656, "Color Box"=u32 16711680) -> (w657:cluster{"String":string, "Color Box":u32})
          }
        }
        n289 = Build Array (concatenate)(w620, w606) -> (w613:cluster{"String":string, "Color Box":u32}[])
        n290 = for {
          tunnel: w613 -> [w633] mode=indexing
          tunnel: [w632] -> w612 mode=indexing
          tunnel: [w631] -> w609
          i -> [w631]
          n291 = Unbundle(w633) -> ("String"=w632:string)  [unwired: 1 out]
        }
        n292 = Concatenate Strings(w612) -> (w611:string)
        n293 = property on="log_box" class="Str"("Text.Text"=w611, "Text.Scroll Position"=w609) -> (error out=w610:errorcluster)  [unwired: 2 in, 1 out]
        n294 = for {
          tunnel: w613 -> [w629] mode=indexing
          shift-right: [w624] -> _
          shift-left: 0 -> [w626]
          shift-right: [w623] -> w608
          shift-left: w610 -> [w627]
          n295 = Unbundle(w629) -> ("String"=w630:string, "Color Box"=w628:u32)
          n296 = String Length(string=w630) -> (length=w625:i32)
          n297 = Add(x=w625, y=w626) -> (x+y=w624:i32)
          n298 = property on="log_box" class="Str"(error in=w627, "Text.Selection End"=w624, "Text.Selection Start"=w626, "Text.FontColor"=w628) -> (error out=w623:errorcluster)  [unwired: 1 in, 1 out]
        }
      }
      frame "Confirm quit" {
        n299 = local read "acquiring?"() -> (w668:bool)
        n300 = local read "logging?"() -> (w662:bool)
        n301 = local read "serving?"() -> (w661:bool)
        n302 = Compound Arithmetic op=OR(w662, w661, w668) -> (w667:bool)
        n303 = case shown="True" w667 {
          tunnel: [TRUE ("Priority Message? (F)") w677] -> w670
          frame False {
          }
          frame True {
            n304 = global read "global_var.vi" "GUI strings"() -> (w676:string[])
            n305 = Index Array(array=w676, index #1=42 ("index")) -> (element #1=w675:string, element #2=w674:string, element #3=w673:string)  [unwired: 2 in]
            n306 = Two Button Dialog(message=w675, 1:w673, 2:w674) -> (T button?=w677:bool)
          }
        }
        n307 = case shown="True" w670 {
          tunnel: w663 -> [w678 w683]
          tunnel: w666 -> [w679 w682]
          tunnel: [w679 w681] -> w665
          tunnel: [w678 w680] -> w664
          frame False {
          }
          frame True {
            n308 = call-poly "que_enqueue_message.vi"("Priority Message? (F)"=TRUE, "error in (no error)"=w682, "Message"="Exit", "Message Queue"=w683) -> ("error out"=w681:errorcluster, "dup Message Queue"=w680:refnum<queue>)  [unwired: 6 in]
          }
        }
      }
      frame "Error", Default {
        # "### If there is an Error in any case, shows it and send Command Exit ###"
        n309 = Variant To Data(error in=w693, type=errorcluster {"status"=FALSE, "code"=0, "source"=""} ("error constant"), Variant=w692) -> (data=w698:errorcluster, error out=w688:errorcluster)
        n310 = call <vilib>:"Simple Error Handler.vi"("error in (no error)"=w698) -> ()  [unwired: 4 in, 5 out]
        n311 = call-poly "que_enqueue_message.vi"("Priority Message? (F)"=TRUE, "Message"="Exit", "Message Queue"=w691) -> ("error out"=w696:errorcluster, "dup Message Queue"=w686:refnum<queue>)  [unwired: 7 in]
        n312 = call <vilib>:"Clear Errors.vi"("error in (no error)"=w688) -> ("error out"=w687:errorcluster)  [unwired: 6 in]
        n313 = Merge Errors(w696, w687) -> (w690:errorcluster)
      }
      frame "Exit" {
        w702 = TRUE ("Priority Message? (F)")
        # "Stops while of UI Message Loop"
        # "Send Exit Message to Loops:\n-Acquisition\n-Server\n-Logging"
        # "Send Stop Event [0]"
        # "Destroy ALL ques"
        n314 = call "uev_fire_user_event_stop.vi"("User Event - Stop"=w713) -> ()  [unwired: 10 in, 1 out]
        n315 = Release Queue(queue=w715, error in (no error)=w714) -> (error out=w709:errorcluster)  [unwired: 1 in, 2 out]
        n316 = Release Queue(queue=w708, error in (no error)=w709) -> (error out=w706:errorcluster)  [unwired: 1 in, 2 out]
        n317 = call-poly "que_enqueue_message.vi"("Priority Message? (F)"=w702, "Message"=w701, "Message Queue"=w711) -> ()  [unwired: 7 in, 2 out]
        n318 = call-poly "que_enqueue_message.vi"("Priority Message? (F)"=w702, "Message"=w701, "Message Queue"=w712) -> ()  [unwired: 7 in, 2 out]
        n319 = call-poly "que_enqueue_message.vi"("Priority Message? (F)"=w702, "Message"=w701, "Message Queue"=w700) -> ()  [unwired: 7 in, 2 out]
        n320 = Release Queue(queue=w707, error in (no error)=w706) -> (error out=w705:errorcluster)  [unwired: 1 in, 2 out]
        n321 = Release Queue(queue=w704, error in (no error)=w705) -> (error out=w703:errorcluster)  [unwired: 1 in, 2 out]
      }
    }
    n322 = call "uev_error_handler_message_handling_loop.vi"("error in (no error)"=w62, "Message Queue"=w51) -> ("dup error in"=w54:errorcluster)  [unwired: 8 in, 1 out]
  }
  n323 = while {
    shift-right: [w723] -> w36
    shift-left: w4 -> [w722]
    tunnel: w19 -> [w721]
    tunnel: [w717] -> w35
    tunnel: w1 -> [w716]
    stop <- w718 stop-if-true
    # "Event Handling Loop"
    n324 = event shown="[5] \"config_files\": Value Change" {
      selector: w722 -> [_ _ _ _ _ _ _ _]
      dyn-events: [_ _ _ _ _ _ _ _] -> w723
      timeout: _ -> [_ _ _ _ _ _ _ _]
      tunnel: w721 -> [_ w727 w744 w763 w792 w797 w803 w805]
      tunnel: [_ w726 w736 w762 w793 w798 w802 _] -> w720
      tunnel: [_ w725 w746 w761 w794 _ w801 _] -> w719
      tunnel: [TRUE ("Discard?") _ _ _ _ _ _ _] -> w718
      tunnel: w716 -> [_ _ w747 _ _ _ _ _]
      event User Event {
        # "Stops While of Event Handling Loop"
        n325 = event-data() -> ()  [unwired: 1 in, 4 out]
      }
      event "stop?": Value Change {
        n326 = event-data() -> ()  [unwired: 1 in, 2 out]
        n327 = case shown="True" "stop?" {
          tunnel: w727 -> [w729 w734]
          tunnel: [w729 w735] -> w726
          tunnel: [_ w732] -> w725
          frame False {
          }
          frame True {
            n328 = To Variant(anything=1) -> (Variant=w730:variant)
            n329 = call-poly "que_enqueue_message.vi"("Message Data"=w730, "Message"="Acquisition stop", "Message Queue"=w734) -> ("error out"=w732:errorcluster, "dup Message Queue"=w735:refnum<queue>)  [unwired: 7 in]
          }
        }
      }
      event Key Down {
        n330 = event-data() -> ("Char"=w745:i16)  [unwired: 1 in, 4 out]
        n331 = To Unsigned Byte Integer(number=w745) -> (unsigned 8bit integer=w741:u8)
        n332 = In Range and Coerce(upper limit=u8 57 ("Char"), x=w741, lower limit=u8 49 ("Char")) -> (In Range?=w738:bool)  [unwired: 1 out]
        n333 = Not(x=w738) -> (.not. x?=w740:bool)
        n334 = Or(x=w740, y="refuse mrk?") -> (x .or. y?=w737:bool)
        n335 = case shown="True" w737 {
          tunnel: w747 -> [w759 _]
          tunnel: [w756 _] -> w746
          tunnel: w741 -> [w755 _]
          tunnel: w744 -> [w753 w760]
          tunnel: [w750 w760] -> w736
          frame False {
            w757 = u8 0  # U8
            n336 = Type Cast(x=w755) -> (*(type *) &x=w752:string)  [unwired: 1 in]
            n337 = global read "global_var.vi" "GUI strings"() -> (w749:string[])
            n338 = Decimal String To Number(string=w752, default (0L)=w757) -> (number=w758:u8)  [unwired: 1 in, 1 out]
            n339 = call "status_string_format.vi"("marker"=w752, "color"=enum16{"Black", "Blue", "Red", "Time"}."Time", "index"=31, "gui_strings"=w749, "Message Queue"=w753) -> ("error out"=w751:errorcluster, "dup Message Queue"=w750:refnum<queue>)  [unwired: 5 in]
            n340 = Enqueue Element(queue=w759, element=w758, error in (no error)=w751) -> (error out=w756:errorcluster)  [unwired: 1 in, 2 out]
          }
          frame True {
          }
        }
      }
      event "log?", "tcp?": Value Change {
        n341 = event-data() -> ("CtlRef"=w765:refnum<vi>, "OldVal"=w764:bool)  [unwired: 1 in, 1 out]
        n342 = Or(x="log?", y="tcp?") -> (x .or. y?=w768:bool)
        n343 = case shown="False" w768 {
          tunnel: "log?" -> [_ w782]
          tunnel: "tcp?" -> [_ w781]
          tunnel: w765 -> [w771 _]
          tunnel: w764 -> [w770 _]
          tunnel: w763 -> [w769 w780]
          tunnel: [w769 w779] -> w762
          tunnel: [_ w778] -> w761
          frame False {
            n344 = global read "global_var.vi" "GUI strings"() -> (w774:string[])
            n345 = property class="Bool (strict)"(reference=w771, "Val(Sgnl)"=w770) -> ()  [unwired: 1 in, 2 out]
            n346 = Index Array(array=w774, index=32) -> (element=w773:string)
            n347 = One Button Dialog(message=w773) -> ()  [unwired: 1 in, 1 out]
          }
          frame True {
            n348 = Build Array(w782, w781) -> (w776:bool[])
            n349 = To Variant(anything=w776) -> (Variant=w775:variant)
            n350 = call-poly "que_enqueue_message.vi"("Message Data"=w775, "Message"="Update booleans", "Message Queue"=w780) -> ("error out"=w778:errorcluster, "dup Message Queue"=w779:refnum<queue>)  [unwired: 7 in]
          }
        }
      }
      event "eeg_txtbox": Value Change {
        n351 = event-data() -> ("NewVal"=w790:string)  [unwired: 1 in, 5 out]
        n352 = Decimal String To Number(string=w790) -> (number=w787:i32)  [unwired: 2 in, 1 out]
        n353 = Increment(x=w787) -> (x+1=w789:i32)
        n354 = To Long Integer(number=w789) -> (32bit integer=w786:i32)
        n355 = Bundle(w786, path "", FALSE) -> (w784:cluster{i32, path, bool})  [unwired: 1 in]
        n356 = To Variant(anything=w784) -> (Variant=w788:variant)
        n357 = call-poly "que_enqueue_message.vi"("Message Data"=w788, "Message"="Device selected", "Message Queue"=w792) -> ("error out"=w794:errorcluster, "dup Message Queue"=w793:refnum<queue>)  [unwired: 7 in]
      }
      event "config_files": Value Change {
        n358 = event-data() -> ("NewVal"=w795:string)  [unwired: 1 in, 5 out]
        n359 = call-poly "que_enqueue_message.vi"("Message Data"=w795, "Message"="Read config", "Message Queue"=w797) -> ("dup Message Queue"=w798:refnum<queue>)  [unwired: 7 in, 1 out]
      }
      event "play?": Value Change {
        n360 = event-data() -> ()  [unwired: 1 in, 1 out]
        n361 = Not(x="play?") -> ()  [unwired: 1 out]
        n362 = call-poly "que_enqueue_message.vi"("Message"="Acquisition start", "Message Queue"=w803) -> ("error out"=w801:errorcluster, "dup Message Queue"=w802:refnum<queue>)  [unwired: 8 in]
      }
      event Panel Close? {
        # "Check if something is running, if not, just exit"
        n363 = event-data() -> ()  [unwired: 1 in, 1 out]
        n364 = call-poly "que_enqueue_message.vi"("Priority Message? (F)"=TRUE, "Message"="Confirm quit", "Message Queue"=w805) -> ()  [unwired: 7 in, 2 out]
        n365 = event-data("Discard?"=TRUE) -> ()  [unwired: 1 in, 1 out]
      }
    }
    n366 = call "uev_error_handler_event_loop.vi"("error in (no error)"=w719, "Message Queue"=w720) -> ("dup error in"=w717:errorcluster)  [unwired: 8 in, 1 out]
  }
  n367 = call "log_loop.vi"("Log queue"=w2, "Message Queues"=w7) -> ("error out"=w13:errorcluster)  [unwired: 9 in]
  n368 = while {
    shift-right: [w812] -> _
    shift-left: 0 ("y") -> [w814]
    tunnel: w4 -> [_]
    stop <- w809 stop-if-true
    # "Server Bar"
    n369 = Wait (ms)(milliseconds to wait=u32 50 ("millisecond multiple")) -> ()  [unwired: 1 out]
    n370 = Increment(x=w814) -> (x+1=w813:i32)
    n371 = Quotient & Remainder(x=w814, y=100) -> (x-y*floor(x/y)=w816:i32)  [unwired: 1 out]
    n372 = local read "stopBars"() -> (w809:bool)
    n373 = Add(x=w816, y=u32 10 ("millisecond multiple")) -> (x+y=w819:u32)
    n374 = Select(t=w813, s="serving?", f=0 ("y")) -> (s? t:f=w812:i32)
    n375 = Bundle(w816, w819) -> (→"srv_bar":cluster{i32, u32})  [unwired: 1 in]
  }
  n376 = while {
    shift-right: [w825] -> _
    shift-left: 0 ("y") -> [w827]
    tunnel: [w821] -> _
    tunnel: w4 -> [w821]
    stop <- w822 stop-if-true
    # "Logging Bar"
    n377 = Wait (ms)(milliseconds to wait=u32 50 ("millisecond multiple")) -> ()  [unwired: 1 out]
    n378 = Increment(x=w827) -> (x+1=w826:i32)
    n379 = Quotient & Remainder(x=w827, y=100) -> (x-y*floor(x/y)=w829:i32)  [unwired: 1 out]
    n380 = local read "stopBars"() -> (w822:bool)
    n381 = Add(x=w829, y=u32 10 ("millisecond multiple")) -> (x+y=w832:u32)
    n382 = Select(t=w826, s="logging?", f=0 ("y")) -> (s? t:f=w825:i32)
    n383 = Bundle(w829, w832) -> (→"log_bar":cluster{i32, u32})  [unwired: 1 in]
  }
  n384 = Unregister For Events(event registration refnum=w36, error in=w35) -> (error out=w34:errorcluster)
  n385 = Merge Errors(w34, w32, w22, w17, w13) -> (w33:errorcluster)
  n386 = call "uev_destroy_user_event_stop.vi"("error in (no error)"=w33, "User Event - Stop"=w31) -> ("error out"=w21:errorcluster)  [unwired: 9 in]
  n387 = Select(t=w20, s=w21, f=w20) -> (s? t:f=w5:bool)
  n388 = local write "stopBars"(w5) -> ()
  n389 = call "mules_exit_exe.vi"("Quit? (T)"=w5) -> ()  [unwired: 2 in]
